vi "Register Tiles Info.vi"(8 "error in (no error)":errorcluster, 9 "Data Message":refnum<class "Data Message.lvclass">, 10 "View Enqueuer":refnum<class "Message Enqueuer.lvclass">, 11 "Project Model in":refnum<class "Project Model.lvclass">) -> (0 "error out":errorcluster, 3 "Project Model out":refnum<class "Project Model.lvclass">)   [LabVIEW 2013, in "Project Model.lvlib" / "Project Model.lvclass"]
uses:
  Project Model.lvclass
  <vilib>/ActorFramework/Message Enqueuer/Message Enqueuer.lvclass
  <vilib>/ActorFrameworkMVC/View Observer/Data Message/Data Message.lvclass
  Project Model.lvclass/Project Model.ctl
  <vilib>/ActorFrameworkMVC/View Observer/View Registry/View Registry.lvclass
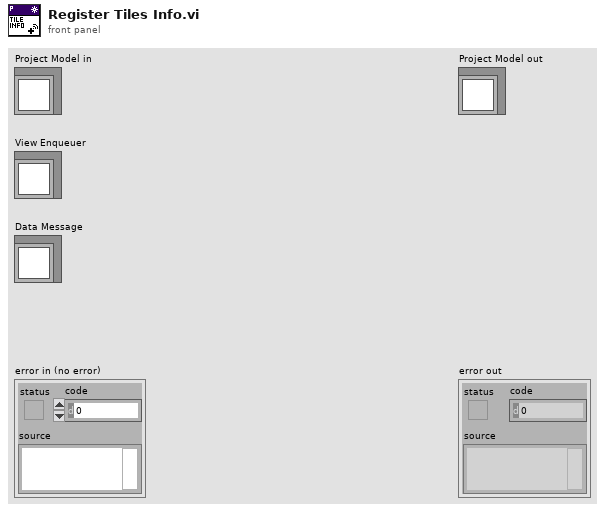
[diagram p1: front panel]
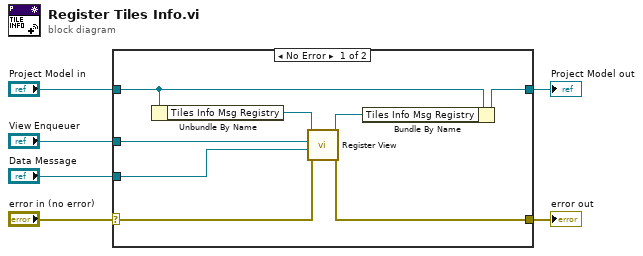
[diagram p0: block diagram]
diagram:
  n1 = case shown="No Error" "error in (no error)" {
    selector: "error in (no error)" -> [w11 w16]
    tunnel: "View Enqueuer" -> [w14 _]
    tunnel: "Project Model in" -> [w13 w15]
    tunnel: "Data Message" -> [w12 _]
    tunnel: [w10 w15] -> w2
    tunnel: [w7 w16] -> w1
    frame No Error {
      n2 = Unbundle By Name(w13) -> ("Tiles Info Msg Registry"=w9:refnum<class "View Registry.lvclass">)
      n3 = call <vilib>:"Register View.vi"("error in (no error)"=w11, "Data Message"=w12, "View Enqueuer"=w14, "View Registry in"=w9) -> ("error out"=w7:errorcluster, "View Registry out"=w8:refnum<class "View Registry.lvclass">)  [unwired: 6 in]
      n4 = Bundle By Name(cluster=w13, "Tiles Info Msg Registry"=w8) -> (w10:refnum<class "Project Model.lvclass">)
    }
    frame Error {
    }
  }
  "error out" <- w1
  "Project Model out" <- w2
